vi "SpecAn BW Set.vi"(0 "VISA In":refnum<visa-resource-name>, 5 "Error In":errorcluster, 6 "Auto RBW (T: Enable)":bool=TRUE, 8 "Manual RBW":i32=3000000 format="%#.5p", 10 "Auto VBW (T: Enable)":bool=TRUE, 12 "Manual VBW":i32=3000001 format="%#.5p") -> (14 "VISA Out":refnum<visa-resource-name>, 19 "Error Out":errorcluster)   [LabVIEW 2015]
uses:
  Controls/FGV Action SpecAn Model.ctl
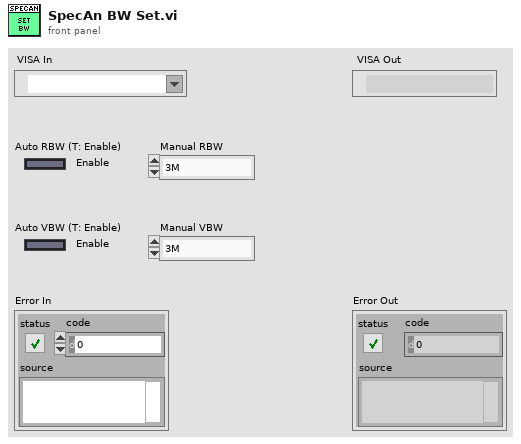
[diagram p1: front panel]
types:
  T1 = typedef "FGV Action SpecAn Model.ctl" = enum16{"Get", "Set"}
  T2 = typedef "SpecAn Model.ctl" = enum16{"E4440", "N9030"}
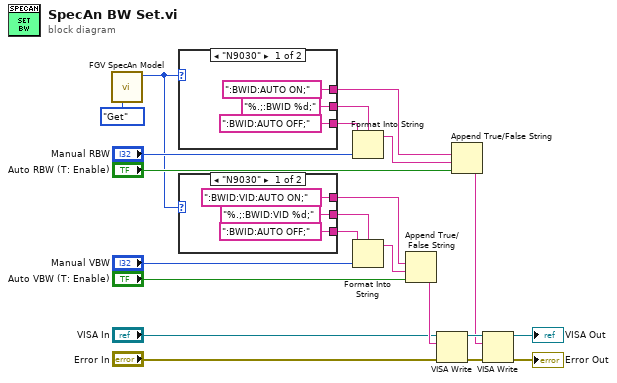
[diagram p0: block diagram]
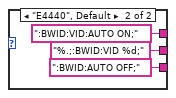
[diagram p2: hidden frame]
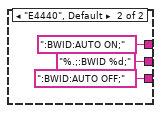
[diagram p3: hidden frame]
diagram:
  n1 = call "FGV SpecAn Model.vi"("Action"=FGV_Action_SpecAn_Model."Get") -> ("SA Model"=w1:T2)  [unwired: 6 in, 1 out]
  n2 = case shown="\"N9030\"" w1 {
    tunnel: [":BWID:AUTO ON;" ("format string") ":BWID:AUTO ON;" ("format string")] -> w20
    tunnel: ["%.;:BWID %d;" ("format string") "%.;:BWID %d;" ("format string")] -> w19
    tunnel: [":BWID:AUTO OFF;" ("format string") ":BWID:AUTO OFF;" ("format string")] -> w10
    frame "N9030" {
    }
    frame "E4440", Default {
    }
  }
  n3 = case shown="\"N9030\"" w1 {
    tunnel: [":BWID:VID:AUTO ON;" ("format string") ":BWID:VID:AUTO ON;" ("format string")] -> w17
    tunnel: ["%.;:BWID:VID %d;" ("format string") "%.;:BWID:VID %d;" ("format string")] -> w16
    tunnel: [":BWID:AUTO OFF;" ("format string") ":BWID:AUTO OFF;" ("format string")] -> w9
    frame "N9030" {
    }
    frame "E4440", Default {
    }
  }
  n4 = Format Into String(format string=w19, initial string=w10, "Manual RBW") -> (resulting string=w18:string)  [unwired: 1 in, 1 out]
  n5 = Format Into String(format string=w16, initial string=w9, "Manual VBW") -> (resulting string=w15:string)  [unwired: 1 in, 1 out]
  n6 = Append True/False String(1:"Auto VBW (T: Enable)", 2:w15, 3:w17) -> (0:w8:string)  [unwired: 1 in]
  n7 = VISA Write(VISA resource name="VISA In", write buffer=w8, error in (no error)="Error In") -> (VISA resource name out=w6:refnum<visa-resource-name>, error out=w5:errorcluster)  [unwired: 1 out]
  n8 = Append True/False String(1:"Auto RBW (T: Enable)", 2:w18, 3:w20) -> (0:w3:string)  [unwired: 1 in]
  n9 = VISA Write(VISA resource name=w6, write buffer=w3, error in (no error)=w5) -> (VISA resource name out=→"VISA Out":refnum<visa-resource-name>, error out=→"Error Out":errorcluster)  [unwired: 1 out]
